vi "corridor_math.vi"(6 "Corridor Width":dbl, 8 "Waypoint Y":dbl, 9 "Waypoint X":dbl, 10 "Irons Range":dbl, 11 "Boat Angle":dbl(slide) scale=0.0..360.0) -> (0 "Y out":dbl, 1 "X out":dbl)   [LabVIEW 2013]
doc: "Tacking math with corridor-shaped boundaries implemented.\n\n23 Jan. 2015\nJoe Sutker"
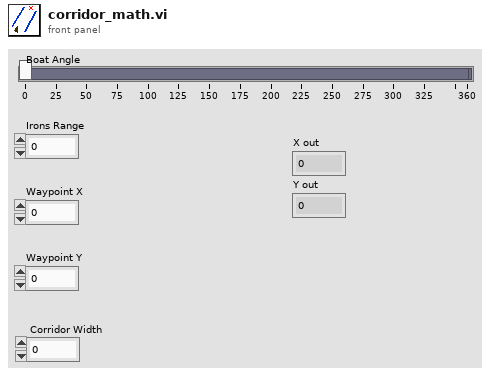
[diagram p1: front panel]
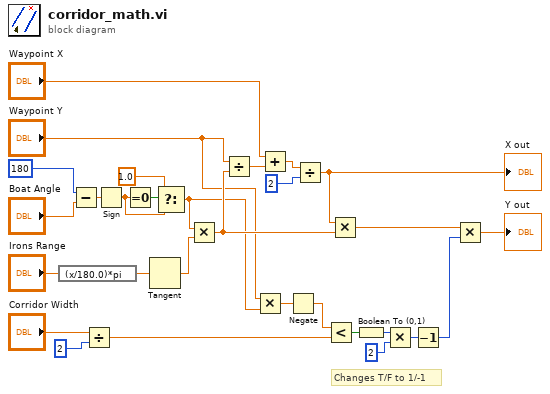
[diagram p0: block diagram]
diagram:
  # "Changes T/F to 1/-1"
  n1 = expression code="(x/180.0)*pi"("Irons Range") -> (w15:dbl)
  n2 = Subtract(x=180, y="Boat Angle") -> (x-y=w29:dbl)
  n3 = Divide(x="Corridor Width", y=2) -> (x/y=w12:dbl)
  n4 = Sign(1:w29) -> (0:w26:dbl)
  n5 = Equal To 0?(x=w26) -> (x = 0?=w28:bool)
  n6 = Tangent(1:w15) -> (0:w25:dbl)
  n7 = Select(t=1.0, s=w28, f=w26) -> (s? t:f=w10:dbl)
  n8 = Multiply(x=w10, y=w25) -> (x*y=w17:dbl)
  n9 = Divide(x="Waypoint Y", y=w17) -> (x/y=w24:dbl)
  n10 = Multiply(x="Waypoint Y", y=w10) -> (x*y=w9:dbl)
  n11 = Add(x="Waypoint X", y=w24) -> (x+y=w22:dbl)
  n12 = Negate(x=w9) -> (-x=w8:dbl)
  n13 = Divide(x=w22, y=2) -> (x/y=w18:dbl)
  "X out" <- w18
  n14 = Less?(x=w8, y=w12) -> (x < y?=w7:bool)
  n15 = Multiply(x=w18, y=w17) -> (x*y=w3:dbl)
  n16 = Boolean To (0,1)(Boolean=w7) -> (0, 1=w6:i16)
  n17 = Multiply(x=w6, y=2) -> (x*y=w4:i32)
  n18 = Decrement(x=w4) -> (x-1=w1:i32)
  n19 = Multiply(x=w3, y=w1) -> (x*y=→"Y out":dbl)
